vi "Get gRPC ID.vi"(11 "OOP Server in":refnum<class "HVC4.lvclass">) -> (2 "gRPC ID":T1, 3 "OOP Server out":refnum<class "HVC4.lvclass">)   [LabVIEW 2019, in "HVC4.lvlib" / "HVC4.lvclass"]
uses:
  HVC4.lvclass
  gRPC lvSupport/Server API/typeDefs/grpcId.ctl
  HVC4.lvclass/HVC4.ctl
  gRPC lvSupport/gprc-lvsupport.lvlib
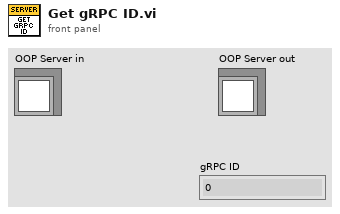
[diagram p1: front panel]
types:
  T1 = typedef "HVC4.lvlib/gprc-lvsupport.lvlib/grpcId.ctl" = u64
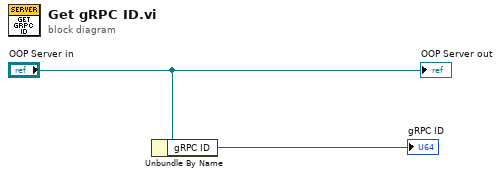
[diagram p0: block diagram]
diagram:
  n1 = Unbundle By Name("OOP Server in") -> ("gRPC ID"=→"gRPC ID":T1)
  "OOP Server out" <- "OOP Server in"
